vi "Launch NIVS and get Ref.vi"(8 "error in (no error)":errorcluster) -> (0 "error out":errorcluster, 3 "WorkspaceManager":T1)   [LabVIEW 2020]
uses:
  <vilib>/NI VeriStand/Execution/Workspace/WorkspaceAPI.ctl
  NationalInstruments.VeriStand.ClientAPI
  <vilib>/registry/registry.llb/Registry SAM.ctl
  <vilib>/registry/registry.llb/Read Registry Value Simple STR.vi
  <vilib>/NI VeriStand/Execution/Workspace/NI_VS Workspace ExecutionAPI.lvlib
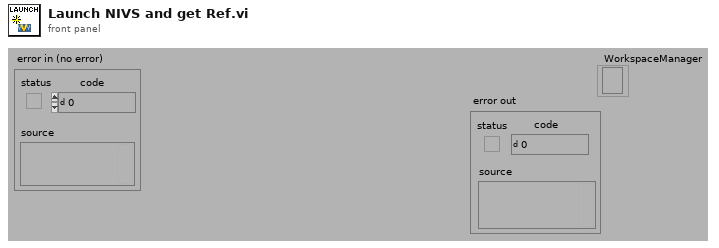
[diagram p1: front panel]
types:
  T1 = typedef "NI_VS Workspace ExecutionAPI.lvlib/WorkspaceAPI.ctl" = refnum<k24>
  T2 = typedef "Registry SAM.ctl" = enum32{"KEY_QUERY_VALUE", "KEY_SET_VALUE", "KEY_CREATE_SUB_KEY", "KEY_ENUMERATE_SUB_KEYS", "KEY_NOTIFY", "KEY_CREATE_LINK", "KEY_READ", "KEY_WRITE", "KEY_ALL_ACCESS", "KEY_READ | KEY_WRITE"}
  T3 = typedef "Registry refnum.ctl" = refnum<k1>
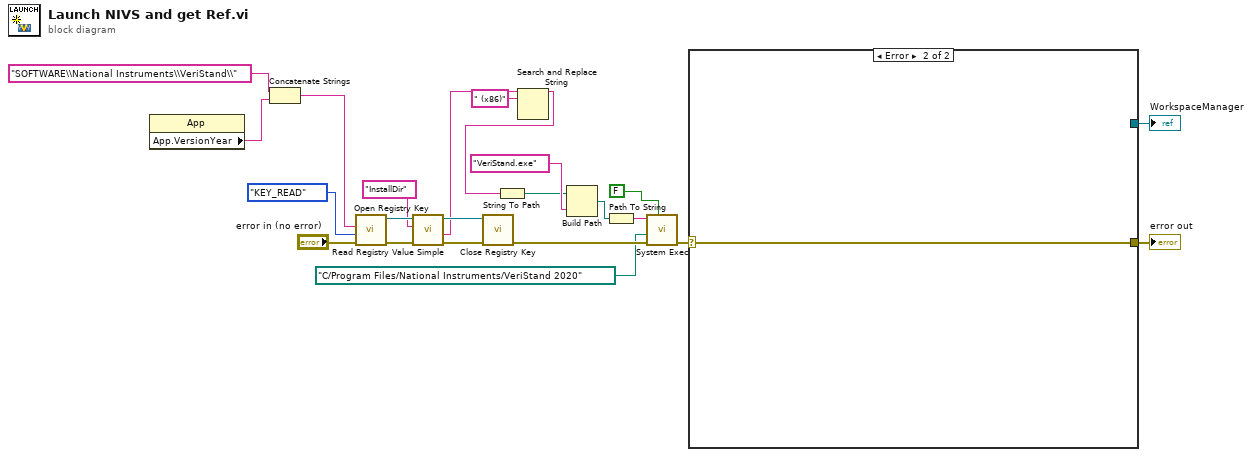
[diagram p0: block diagram]
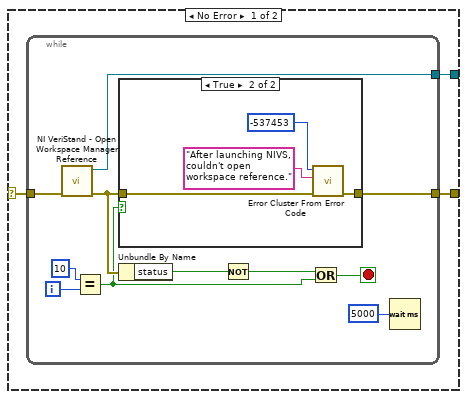
[diagram p2: hidden frame]
diagram:
  n1 = property class="App"() -> ("App.VersionYear"=w6:string)  [unwired: 2 in, 2 out]
  n2 = Concatenate Strings("SOFTWARE\\National Instruments\\VeriStand\\" ("subkey"), w6) -> (w7:string)
  n3 = call <vilib>:"Open Registry Key.vi"("error in (no error)"="error in (no error)", "security access mask (KEY_READ | KEY_WRITE)"=Registry_SAM."KEY_READ", "subkey"=w7) -> ("error out"=w21:errorcluster, "refnum out"=w20:T3)  [unwired: 7 in]
  n4 = call-poly <vilib>:"Read Registry Value Simple.vi"("error in (no error)"=w21, "value"="InstallDir", "refnum"=w20) -> ("error out"=w17:errorcluster, "String/Binary data"=w3:string, "refnum out"=w16:T3)  [unwired: 3 in, 1 out]
  n5 = call <vilib>:"Close Registry Key.vi"("error in (no error)"=w17, "refnum"=w16) -> ("error out"=w15:errorcluster)  [unwired: 5 in]
  n6 = Search and Replace String(input string=w3, search string=" (x86)") -> (result string=w1:string)  [unwired: 6 in, 3 out]
  n7 = String To Path(string=w1) -> (path=w12:path)
  n8 = Build Path(base path=w12, name or relative path="VeriStand.exe") -> (appended path=w14:path)
  n9 = Path To String(path=w14) -> (string=w13:string)
  n10 = call <vilib>:"System Exec.vi"("wait until completion? (T)"=FALSE, "error in (no error)"=w15, "working directory"=path "C:/Program Files/National Instruments/VeriStand 2020", "command line"=w13) -> ("error out"=w10:errorcluster)  [unwired: 4 in, 3 out]
  n11 = case shown="Error" w10 {
    selector: w10 -> [w26 w43]
    tunnel: [w25 w43] -> w9
    tunnel: [w24 _] -> w8
    frame No Error {
      n12 = while {
        tunnel: [w32] -> w24
        tunnel: w26 -> [w33]
        tunnel: [w34] -> w25
        i -> [w36]
        stop <- w27 stop-if-true
        n13 = call <vilib>:"NI VeriStand - Open Workspace Manager Reference.vi"("error in (no error)"=w33) -> ("error out"=w31:errorcluster, "WorkspaceManager"=w32:T1)  [unwired: 9 in]
        n14 = Equal?(x=10, y=w36) -> (x = y?=w28:bool)
        n15 = case shown="True" w28 {
          tunnel: [w38 w41] -> w34
          tunnel: w31 -> [w38 w42]
          frame False {
          }
          frame True {
            n16 = call <vilib>:"Error Cluster From Error Code.vi"("error in (no error)"=w42, "error message (\"\")"="After launching NIVS, couldn't open workspace reference." ("error message (\"\")"), "error code (0)"=-537453) -> ("error out"=w41:errorcluster)  [unwired: 6 in]
          }
        }
        n17 = Unbundle By Name(w31) -> ("status"=w30:bool)
        n18 = Not(x=w30) -> (.not. x?=w29:bool)
        n19 = Or(x=w29, y=w28) -> (x .or. y?=w27:bool)
        n20 = Wait (ms)(milliseconds to wait=u32 5000) -> ()  [unwired: 1 out]
      }
    }
    frame Error {
    }
  }
  "error out" <- w9
  "WorkspaceManager" <- w8
